vi "DraggingDresser.vi"() -> ()   [LabVIEW 2015]
panel:
  out "Force":dbl[](array[numeric])
  out "Angle for Minimum Force":i32 format="%.1f"
  in  "Coefficient of Kinetic Friction":dbl format="%.1f"
  out "Awesome Graph":dbl[](graph)
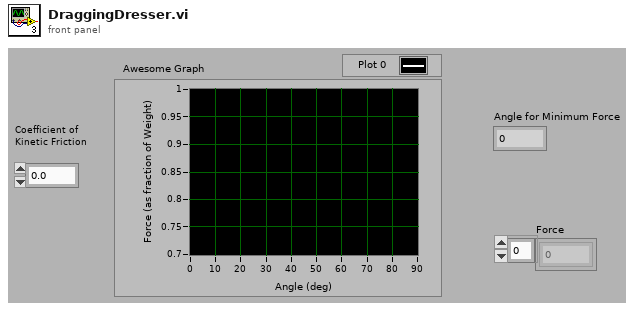
[diagram p1: front panel]
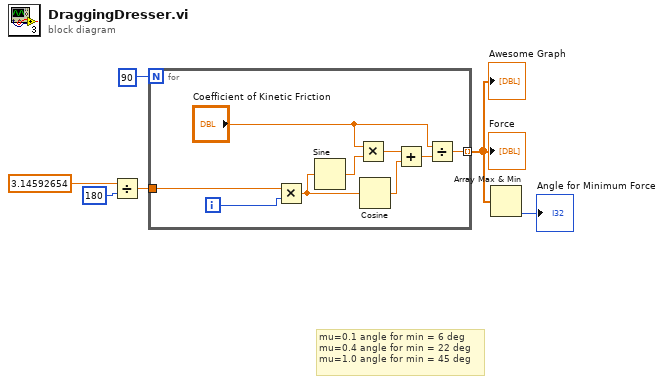
[diagram p0: block diagram]
diagram:
  # "mu=0.1 angle for min = 6 deg\nmu=0.4 angle for min = 22 deg\nmu=1.0 angle for min = 45 deg"
  n1 = Divide(x=3.14592654, y=180) -> (x/y=w1:dbl)
  n2 = for {
    N: 90 -> [_]
    tunnel: [w10] -> w4 mode=indexing
    tunnel: w1 -> [w8]
    i -> [w9]
    n3 = Multiply(x=w8, y=w9) -> (x*y=w7:dbl)
    n4 = Sine(x=w7) -> (sin(x)=w15:dbl)
    n5 = Multiply(x="Coefficient of Kinetic Friction", y=w15) -> (x*y=w14:dbl)
    n6 = Cosine(x=w7) -> (cos(x)=w13:dbl)
    n7 = Add(x=w14, y=w13) -> (x+y=w12:dbl)
    n8 = Divide(x="Coefficient of Kinetic Friction", y=w12) -> (x/y=w10:dbl)
  }
  "Awesome Graph" <- w4
  "Force" <- w4
  n9 = Array Max & Min(array=w4) -> (min index (indices)=→"Angle for Minimum Force":i32)  [unwired: 3 out]
